vi "Total Hold Data.vi"(10 "Contol\nPoint\nSuffix":T1) -> (3 "Data":dbl[](array[numeric]))   [LabVIEW 2009]
uses:
  NTCP Client/Control Point Suffix.ctl
  Data Access Objects/Metadata/DAO Actions.ctl
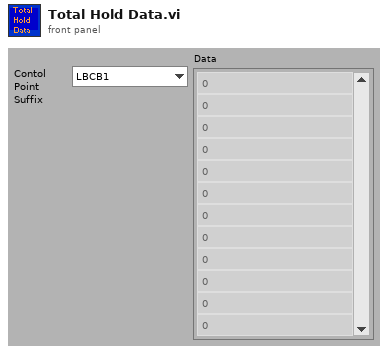
[diagram p1: front panel]
types:
  T1 = typedef "Control Point Suffix.ctl" = enum16{"LBCB1", "LBCB2", "ExternalSensors"}
  T2 = typedef "DAO Actions.ctl" = enum16{"Init", "Get", "Set"}
  T3 = typedef "LBCB Number.ctl" = enum16{"LBCB1", "LBCB2"}
  T4 = typedef "Cartesian Data Type.ctl" = cluster{"Displacements":dbl[], "Forces":dbl[], "Displacement Commands":dbl[]}
  T5 = typedef "Actuator DataType.ctl" = cluster{"LVDTs":dbl[], " Commands":dbl[], "Load Cells":dbl[], "Servo":dbl[]}
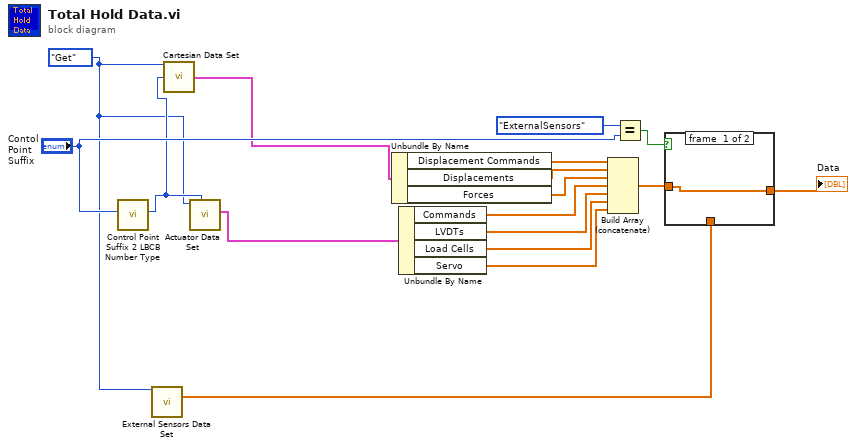
[diagram p0: block diagram]
diagram:
  w1 = DAO_Actions."Get" ("DAO Actions")
  n1 = call "Control Point Suffix 2 LBCB Number Type.vi"("Contol\nPoint\nSuffix"="Contol\nPoint\nSuffix") -> ("LBCB Number"=w3:T3)  [unwired: 10 out]
  n2 = call "External Sensors Data Set.vi"("DAO Actions"=w1) -> ("Hold Data Out"=w5:dbl[])  [unwired: 11 in, 3 out]
  n3 = call "Cartesian Data Set.vi"("DAO Actions"=w1, "LBCB Selected"=w3) -> ("Cartesian Data Hold Data Out"=w2:T4)  [unwired: 3 in, 10 out]
  n4 = call "Actuator Data Set.vi"("Selected LBCB"=w3, "DAO Actions"=w1) -> ("Actuator Data Out"=w4:T5)  [unwired: 3 in, 6 out]
  n5 = Unbundle By Name(w2) -> ("Displacement Commands"=w17:dbl[], "Displacements"=w16:dbl[], "Forces"=w15:dbl[])
  n6 = Unbundle By Name(w4) -> ("Commands"=w14:dbl[], "LVDTs"=w13:dbl[], "Load Cells"=w12:dbl[], "Servo"=w11:dbl[])
  n7 = Build Array (concatenate)(w17, w16, w15, w14, w13, w12, w11) -> (w10:dbl[])
  n8 = Equal?(x=Control_Point_Suffix."ExternalSensors", y="Contol\nPoint\nSuffix") -> (x = y?=w8:bool)
  n9 = case shown="True" w8 {
    tunnel: w10 -> [w18 _]
    tunnel: [w18 w19] -> w9
    tunnel: w5 -> [_ w19]
    frame #0 {
    }
    frame #1 {
    }
  }
  "Data" <- w9
